vi "Write DelayedActivation.vi"(8 "error in (no error)":errorcluster, 10 "DelayedActivation":bool, 11 "CS++ControllerActor in":refnum<class "CS++ControllerActor.lvclass">) -> (0 "error out":errorcluster, 3 "CS++ControllerActor out":refnum<class "CS++ControllerActor.lvclass">)   [LabVIEW 2014, in "CS++ControllerActor.lvlib" / "CS++ControllerActor.lvclass"]
uses:
  CS++ControllerActor.lvclass
  CS++ControllerActor.lvclass/CS++ControllerActor.ctl
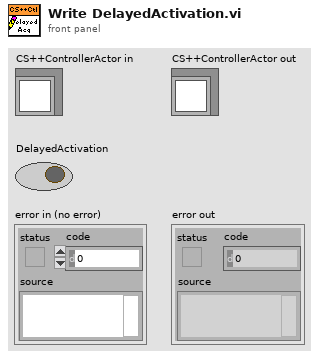
[diagram p1: front panel]
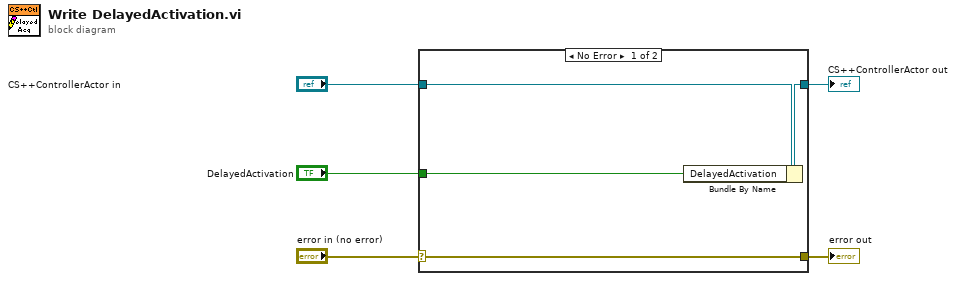
[diagram p0: block diagram]
diagram:
  n1 = case shown="No Error" "error in (no error)" {
    selector: "error in (no error)" -> [w9 w10]
    tunnel: [w9 w10] -> w4
    tunnel: [w7 w11] -> w2
    tunnel: "CS++ControllerActor in" -> [w8 w11]
    tunnel: "DelayedActivation" -> [w6 _]
    frame No Error {
      n2 = Bundle By Name(cluster=w8, "DelayedActivation"=w6) -> (w7:refnum<class "CS++ControllerActor.lvclass">)
    }
    frame Error {
    }
  }
  "error out" <- w4
  "CS++ControllerActor out" <- w2
